vi "Day1_DI.vi"() -> ()   [LabVIEW 2023]
doc: "This example demonstrates how to acquire a continuous amount of digital data based off of the changes of an external signal across one or many lines on either the rising or falling edges. The change detection lines do not have to be in the task. \n\nFor instructions on how to connect your signals to the DAQ device, refer to your device documentation."
uses:
  <vilib>/Utility/error.llb/DialogType.ctl
  <vilib>/DAQmx/configure/timing.llb/DAQmx Timing (Sample Clock).vi
  <vilib>/DAQmx/read.llb/DAQmx Read (Digital 2D Bool NChan 1Samp NLine).vi
  <vilib>/DAQmx/create/channels.llb/DAQmx Create Channel (DI-Digital Input).vi
panel:
  out "data":bool[][](array[boolean])
  in  "Stop":bool
  in  "Line(s)":tag="Dev1/port0/line0:7"
  # "Channel Settings"
  # "Acquired Data"
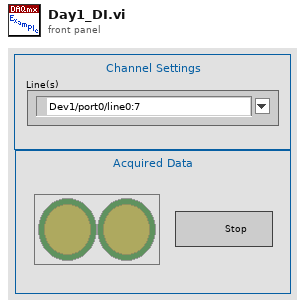
[diagram p1: front panel]
types:
  T1 = typedef "DialogType.ctl" = u16
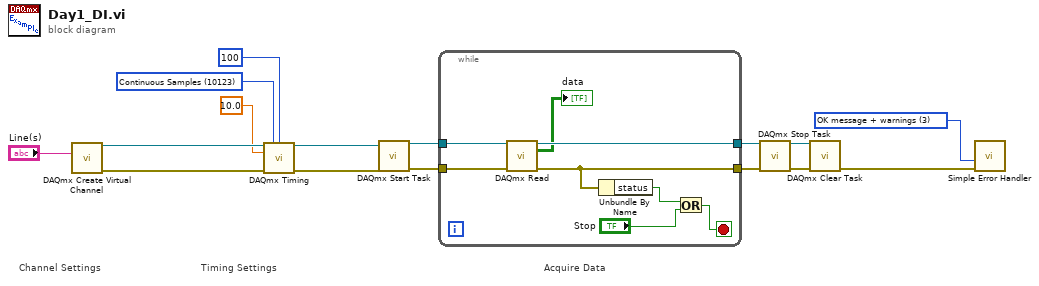
[diagram p0: block diagram]
diagram:
  w14 = 10123 items=["Finite Samples"=10178, "Continuous Samples"=10123, "Hardware Timed Single Point"=12522] ("Sample Mode")
  w3 = T1 3 items=["no dialog", "OK message", "continue or stop message", "OK message + warnings", "continue/stop + warnings"] ("type of dialog (OK msg:1)")
  # "Timing Settings"
  # "Acquire Data"
  # "Channel Settings"
  n1 = call-poly <vilib>:"DAQmx Create Virtual Channel.vi"("lines"="Line(s)") -> ("task out"=w13:refnum<k21>, "error out"=w12:errorcluster)  [unwired: 13 in]
  n2 = call-poly <vilib>:"DAQmx Timing.vi"("task/channels in"=w13, "sample mode"=w14, "samples per channel"=100, "rate"=10.0, "error in"=w12) -> ("task out"=w11:refnum<k21>, "error out"=w10:errorcluster)  [unwired: 9 in]
  n3 = call <vilib>:"DAQmx Start Task.vi"("task/channels in"=w11, "error in"=w10) -> ("task out"=w8:refnum<k21>, "error out"=w9:errorcluster)  [unwired: 12 in]
  n4 = while {
    tunnel: [w24] -> w5
    tunnel: [w21] -> w4
    tunnel: w9 -> [w23]
    tunnel: w8 -> [w22]
    stop <- w18 stop-if-true
    n5 = call-poly <vilib>:"DAQmx Read.vi"("task/channels in"=w22, "error in"=w23) -> ("task out"=w24:refnum<k21>, "data"=→"data":bool[][], "error out"=w21:errorcluster)  [unwired: 11 in]
    n6 = Unbundle By Name(w21) -> ("status"=w20:bool)
    n7 = Or(x=w20, y="Stop") -> (x .or. y?=w18:bool)
  }
  n8 = call <vilib>:"DAQmx Stop Task.vi"("task/channels in"=w5, "error in"=w4) -> ("task out"=w7:refnum<k21>, "error out"=w6:errorcluster)  [unwired: 12 in]
  n9 = call <vilib>:"DAQmx Clear Task.vi"("task in"=w7, "error in"=w6) -> ("error out"=w16:errorcluster)  [unwired: 13 in]
  n10 = call <vilib>:"Simple Error Handler.vi"("type of dialog (OK msg:1)"=w3, "error in (no error)"=w16) -> ()  [unwired: 3 in, 5 out]
